vi "fake main magnet module.vi"(8 "Queue to UI":T10, 11 "Module queue":T10) -> ()   [LabVIEW 2022 SP3, in "Magnet module.lvlib"]
doc: "Magnet module controls: power supply unit (PSU/SMS) and temperature monitor (TM/LSC218).\nPSU controls mainly: switch heater and ramping of current which runs throught coil.\nTM controls temperature of switch, coil and cryostat.\nMessage for magnet is a cluster that contains: {(enum) Command , (variant) Data}\nFor simplifieing of documentation, the Command is noted as a name of instruction, and Data is represented by a requered datatype (mostly cluster) name.\nCommands:\nInitialize(Magnet Config Constants) - Sugesstion: Load configuration constants from configuration file.\nSet field (Set field{B, R, cr}) - B-field[T], R-ramp[A/s], cr - custom ramp[bool].\nSwitch mode(mode) - to persistant, or to ramping.\nBlackout() - undone functionality of emergency deenergizing.\nUpdate() - Important! This triggers update of data from instruments. Shoud occure in regular intervals as priority message.\nResponses:\nMagnet initialized ();\nTM revision(temperature monitor revision);\nMagnet init error(error);\nSetting field(Set Field{B, R, cr});\nWarning(string);\nSwitching to(mode);\nUpdate error(error);\nTM update(TM sensors);\nPSU update(PSU data);\nMagnet status();"
uses:
  Magnet module.lvlib
  Messenger service/Data types/Mailbox address.ctl
  <instrlib>/SMS 120/Public/PSU Status.ctl
  ctl/Cryostat temperature sensors.ctl
  ctl/Overall status.ctl
  ctl/SetField data.ctl
  ctl/Magnet mode public.ctl
  ctl/Actual magnet state.ctl
  ctl/Magnet mode.ctl
  ctl/RampingOutput.ctl
  ctl/Magnet config constants.ctl
  ctl/MagnetStates.ctl
  Messenger service/Data types/Module name.ctl
  ctl/TM Revision.ctl
  ctl/MSG to magnet.ctl
  ctl/Magnet Orders.ctl
  <instrlib>/SMS 120/Cryogenic Ltd SMSXXX.lvlib
  Messenger service/MessengerLib.lvlib
panel:
  in  "LSC218 sensors":T1={"First stage A [K]"=35.0, "Second stage A [K]"=4.0, "Firs stage B [K]"=33.0, "Second stage B [K]"=3.0, "Inner magnet [K]"=3.0, "Outer Magnet [K]"=3.5, "Switch [K]"=3.6, "Support plate [K]"=8.0, "Time stamp"=0.0} {"Time stamp" format="%<%H:%M:%S%2u\n%Y/%m/%d>T"}
  out "Magnet Constants":T2={"Switch resistant [K]"=5.0, "Switch superconducting [K]"=4.0, "First stage critical temperature [K]"=50.0, "Second stage critical temperature [K]"=5.0, "Inner magnet critical temperature [K]"=6.0, "Outer magnet critical temperature [K]"=5.0, "Field Constant [T/A]"=0.14911, "Maximum Current [A]"=107.3, "Maximum field [T]"=16.0, "Maximum source ramp [A/s]"=0.5, "Source precision [T]"=2e-05, "Ramp limits [A/s]"=[0.0506, 0.038, 0.0285, 0.0213, 0.0104], "Field limits [T]"=[3.0, 9.6, 13.3, 15.5, 16.0], "SMS"="", "LSC218"=""}
  out "Overall status":T3={"Desired"={"Field [T]"=0.0, "Ramp [T/s]"=0.0, "Custom Ramp?"=TRUE, "Mode"=enum."Persistant"}, "Actual"={"Mode"=enum."Persistant", "Ramping output"=enum."At Target", "Ready for change"=FALSE, "Switch heater"=FALSE, "Cooler Overheat"=FALSE, "Coil overheat"=FALSE, "Energized"=FALSE, "Output [T]"=0.0, "Field [T]"=0.0, "Ramp[T/s]"=0.0, "Switch\ntemperature [K]"=1.0, "Voltage [V]"=0.0, "Current direction"=FALSE}}
  out "Temperatures":T1[](array[typedef]) {"Time stamp" format="%<%H:%M:%S%2u\n%Y/%m/%d>T"}
  out "PSU Status Out":T9 {"Trip Current" format="%.3f"; "Trip Field" format="%.4f"; "Voltage" format="%.2f"; "Field Constant" format="%.6f"; "MID Setpoint (T)" format="%.4f"; "MID Setpoint (A)" format="%.3f"; "MAX Setpoint (T)" format="%.4f"; "MAX Setpoint (A)" format="%.3f"; "Heater Voltage" format="%.2f"; "V Limit (V)" format="%.2f"; "Ramp Rate (A/s)" format="%.3f"; "Output (A)" format="%.3f"; "Output (T)" format="%.4f"; "Persistent Current" format="%.3f"; "Persistent Field" format="%.4f"}
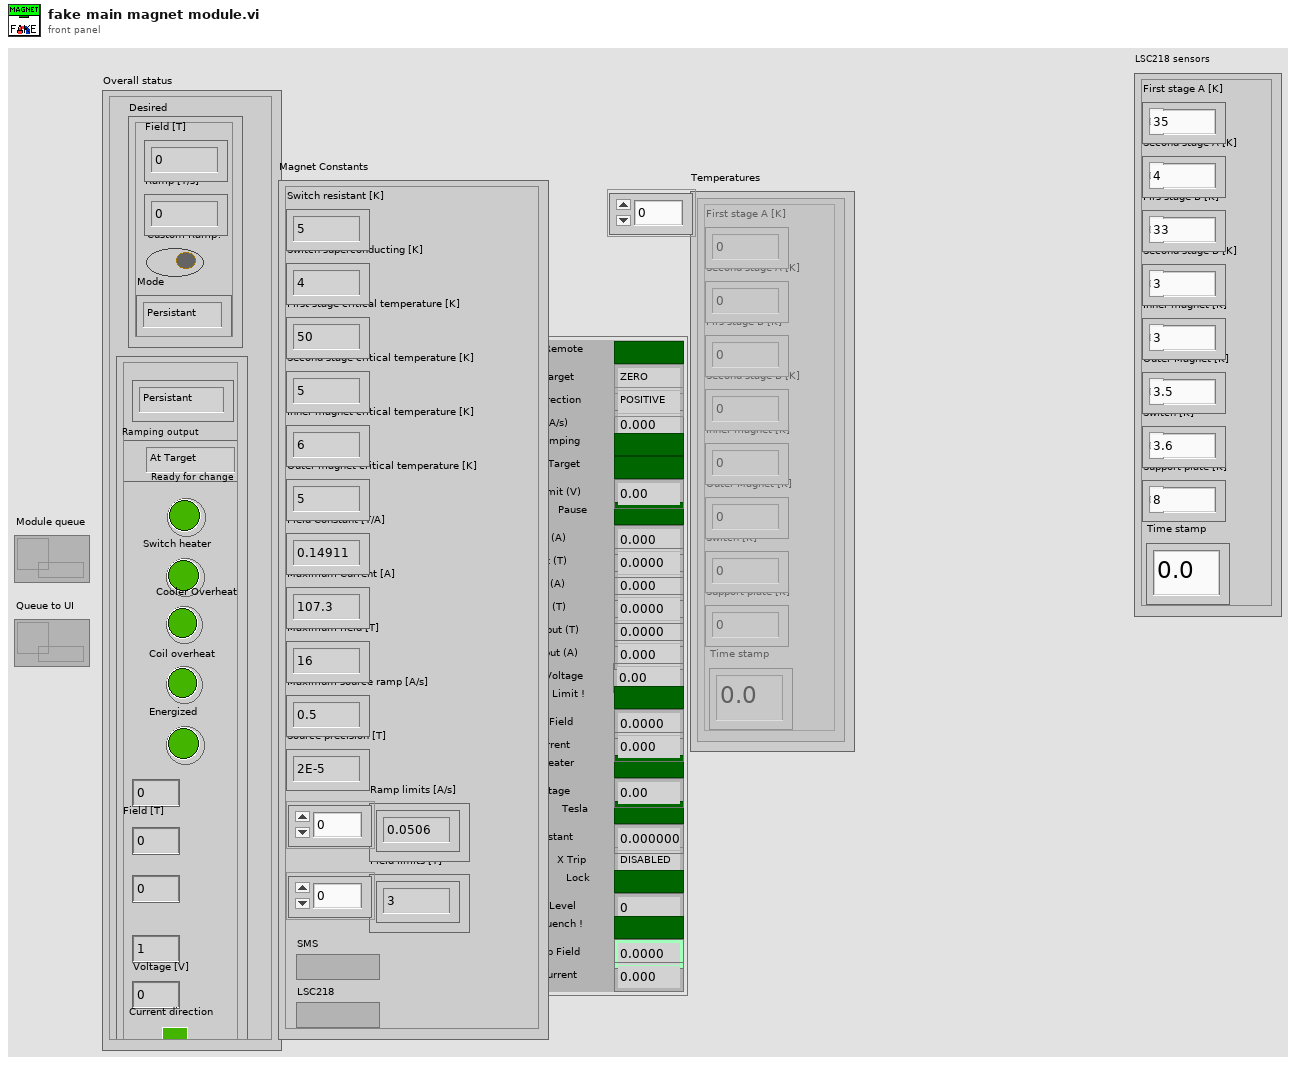
[diagram p1: front panel]
types:
  T1 = typedef "Magnet module.lvlib/Cryostat temperature sensors.ctl" = cluster{"First stage A [K]":dbl, "Second stage A [K]":dbl, "Firs stage B [K]":dbl, "Second stage B [K]":dbl, "Inner magnet [K]":dbl, "Outer Magnet [K]":dbl, "Switch [K]":dbl, "Support plate [K]":dbl, "Time stamp":dbl}
  T2 = typedef "Magnet module.lvlib/Magnet config constants.ctl" = cluster{"Switch resistant [K]":dbl, "Switch superconducting [K]":dbl, "First stage critical temperature [K]":dbl, "Second stage critical temperature [K]":dbl, "Inner magnet critical temperature [K]":dbl, "Outer magnet critical temperature [K]":dbl, "Field Constant [T/A]":dbl, "Maximum Current [A]":dbl, "Maximum field [T]":dbl, "Maximum source ramp [A/s]":dbl, "Source precision [T]":dbl, "Ramp limits [A/s]":dbl[], "Field limits [T]":dbl[], "SMS":refnum<visa-resource-name>, "LSC218":refnum<visa-resource-name>}
  T3 = typedef "Magnet module.lvlib/Overall status.ctl" = cluster{"Desired":T4, "Actual":T6}
  T4 = typedef "Magnet module.lvlib/SetField data.ctl" = cluster{"Field [T]":dbl, "Ramp [T/s]":dbl, "Custom Ramp?":bool, "Mode":T5}
  T5 = typedef "Magnet module.lvlib/Magnet mode public.ctl" = enum16{"Persistant", "Ramping"}
  T6 = typedef "Magnet module.lvlib/Actual magnet state.ctl" = cluster{"Mode":T7, "Ramping output":T8, "Ready for change":bool, "Switch heater":bool, "Cooler Overheat":bool, "Coil overheat":bool, "Energized":bool, "Output [T]":dbl, "Field [T]":dbl, "Ramp[T/s]":dbl, "Switch\ntemperature [K]":dbl, "Voltage [V]":dbl, "Current direction":bool}
  T7 = typedef "Magnet module.lvlib/Magnet mode.ctl" = enum16{"Persistant", "Switching", "Ramping", "Quenched"}
  T8 = typedef "Magnet module.lvlib/RampingOutput.ctl" = enum16{"At Target", "Go up", "Go down"}
  T9 = typedef "Cryogenic Ltd SMSXXX.lvlib/PSU Status.ctl" = cluster{"Ramp Target":enum16{"ZERO", "MID", "MAX"}, "Pause":bool, "Switch Heater":bool, "Persistent Field":dbl, "Persistent Current":dbl, "Tesla":bool, "Output (T)":dbl, "Output (A)":dbl, "X Trip":enum16{"DISABLED", "ENABLED", "ACTIVE"}, "Ramp Rate (A/s)":dbl, "V Limit (V)":dbl, "Heater Voltage":dbl, "MAX Setpoint (A)":dbl, "MAX Setpoint (T)":dbl, "MID Setpoint (A)":dbl, "MID Setpoint (T)":dbl, "Lock":bool, "Field Constant":dbl, "Remote":bool, "Direction":enum16{"POSITIVE", "NEGATIVE", "OPEN", "UNIPOLAR"}, "Helium Level":u16, "Quench !":bool, "Voltage":dbl, "V Limit !":bool, "Ramping":bool, "At Target":bool, "Trip Field":dbl, "Trip Current":dbl}
  T10 = typedef "MessengerLib.lvlib/Mailbox address.ctl" = refnum<queue>
  T11 = typedef "Magnet module.lvlib/MagnetStates.ctl" = enum16{"Initialize", "Regular check", "Check message", "Set Field", "Switch mode", "Restart", "Stop"}
  T12 = typedef "Magnet module.lvlib/MSG to magnet.ctl" = cluster{"Command":T13, "Data":variant}
  T13 = typedef "Magnet module.lvlib/Magnet Orders.ctl" = enum16{"Ignore", "Connect", "Update", "Switch mode", "Set field", "Stop ramping", "Equalize output", "Zero output", "Flip polarity", "Blackout", "Set timer", "Eval temperatures", "Disconnect"}
  T14 = typedef "Module name.ctl" = enum16{"Emty", "Magnet", "VTI", "Excitation", "Servo", "Acquisition", "Rotator", "Digitizer", "SMU2450", "Carousel", "Multimeter", "Tmp monitor", "Power monitor"}
  T15 = typedef "Magnet module.lvlib/TM Revision.ctl" = cluster{"Instr Serial Number":string, "Instr Driver Revision":string, "Instr Firmware Revision":string, "Instr Model Number":string}
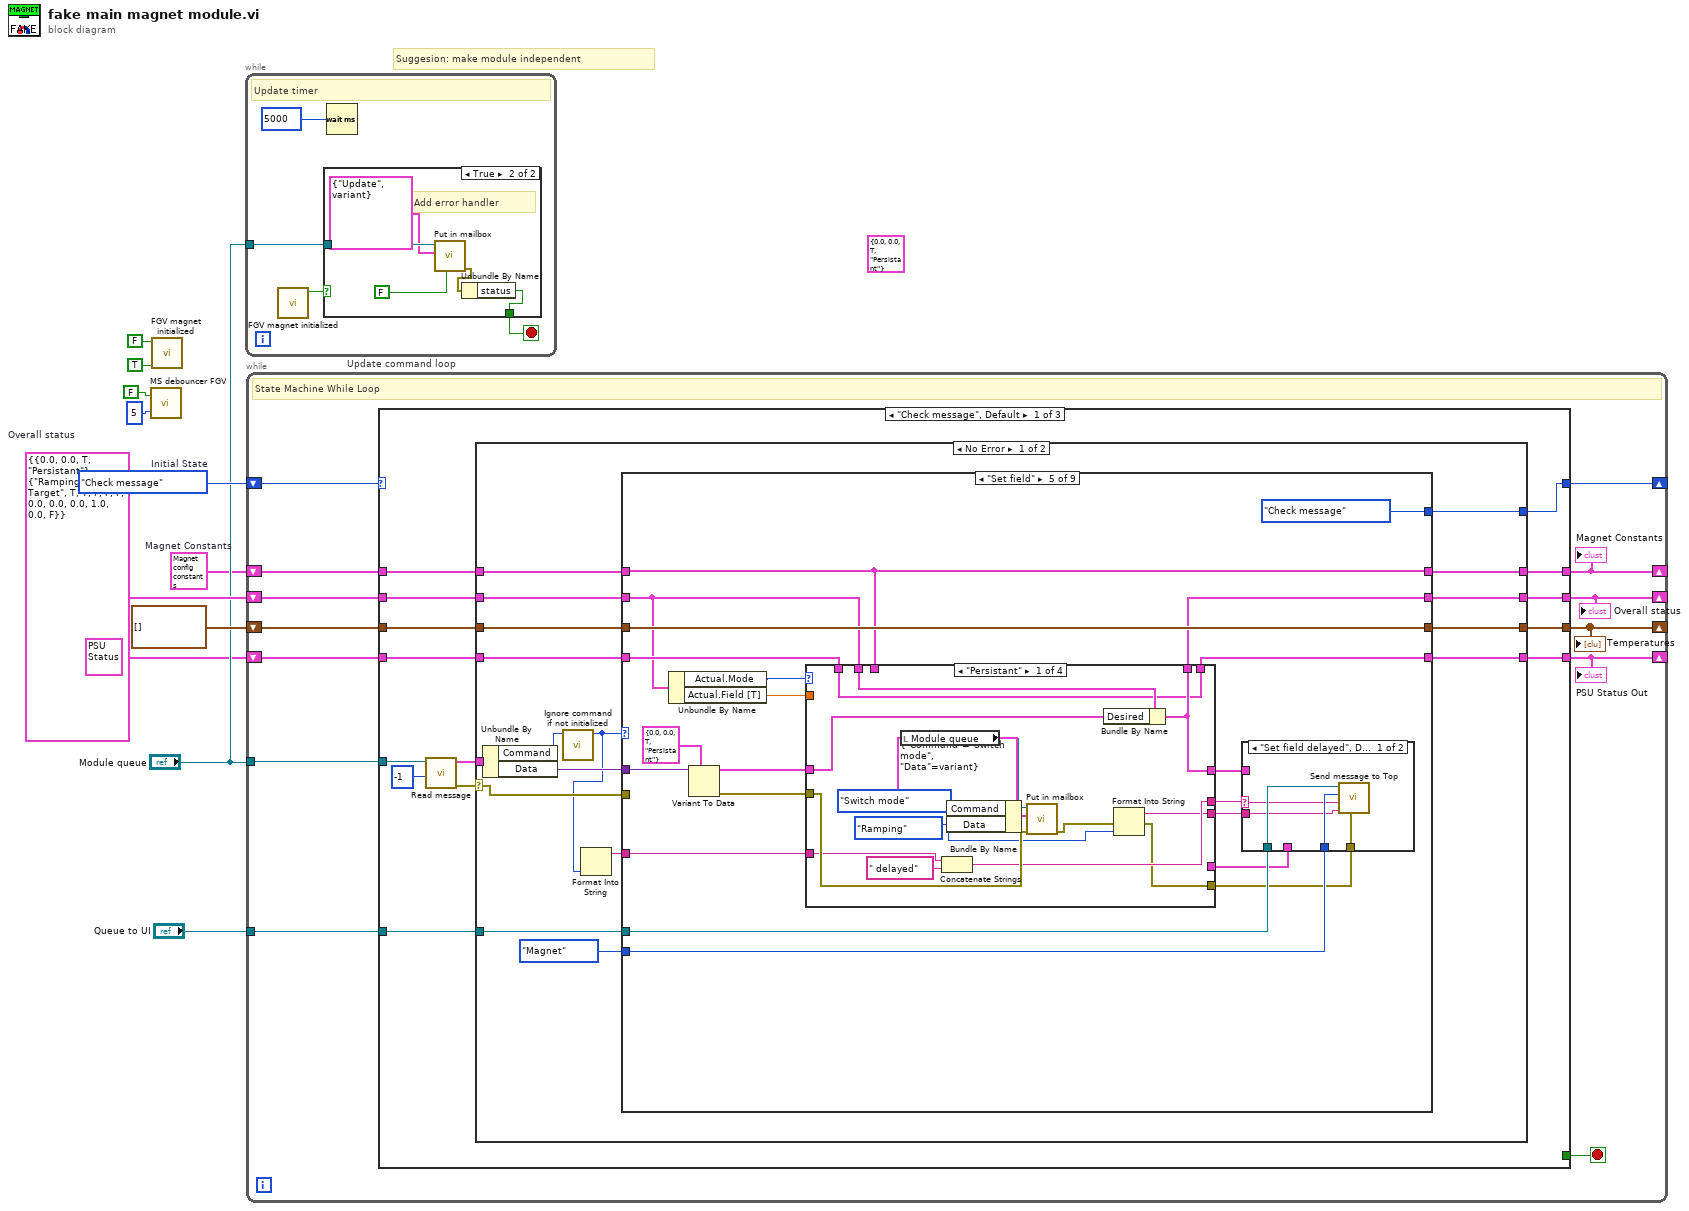
[diagram p0: block diagram]
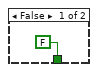
[diagram p2: hidden frame]
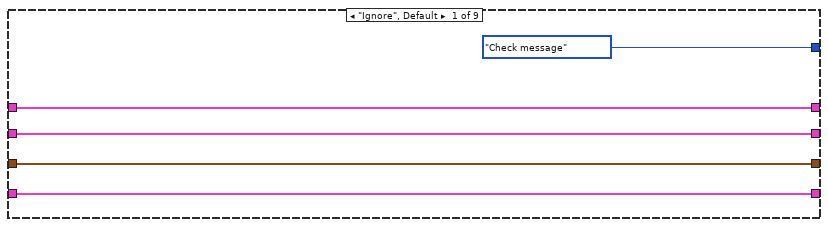
[diagram p3: hidden frame]
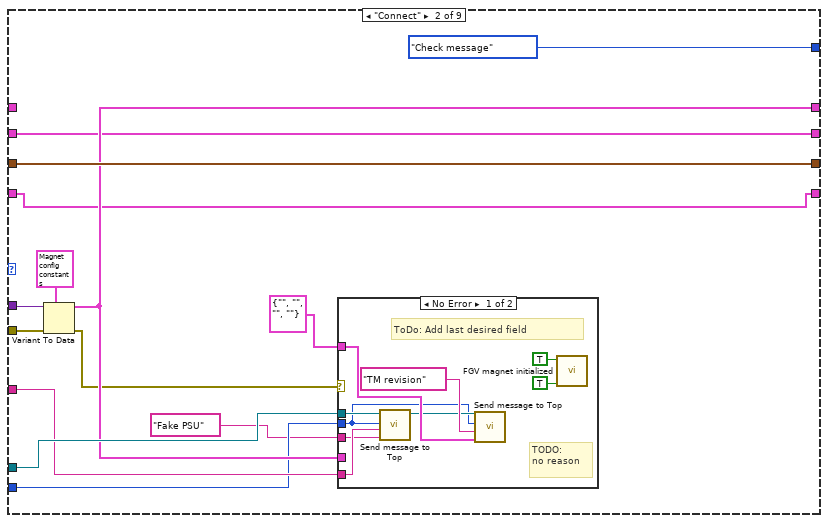
[diagram p4: hidden frame]
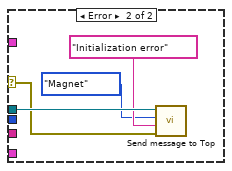
[diagram p5: hidden frame]
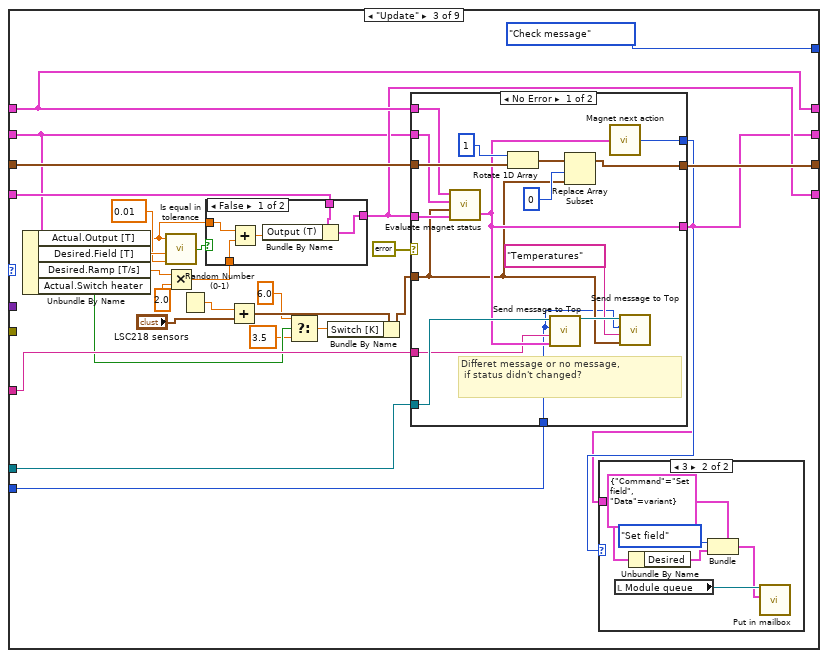
[diagram p6: hidden frame]
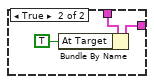
[diagram p8: hidden frame]
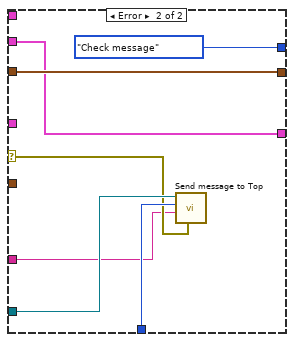
[diagram p9: hidden frame]
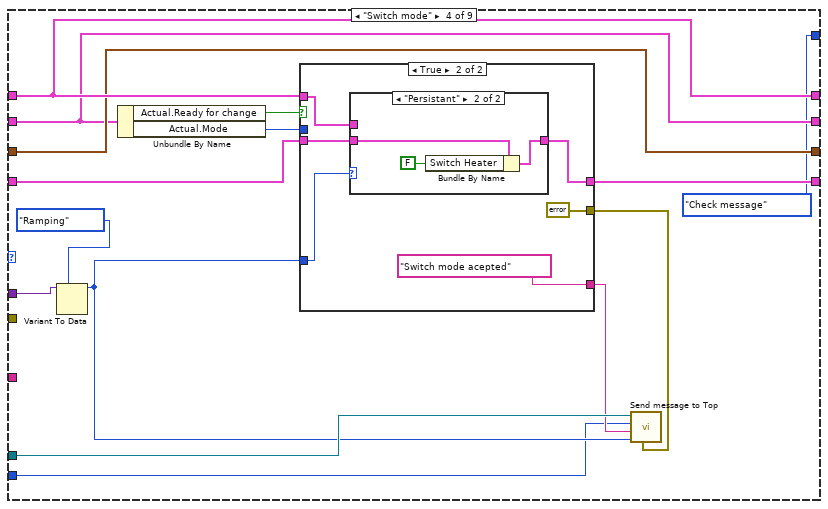
[diagram p10: hidden frame]
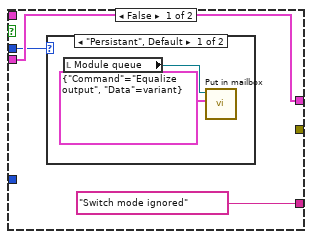
[diagram p11: hidden frame]
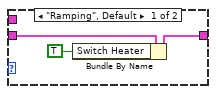
[diagram p13: hidden frame]
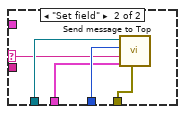
[diagram p14: hidden frame]
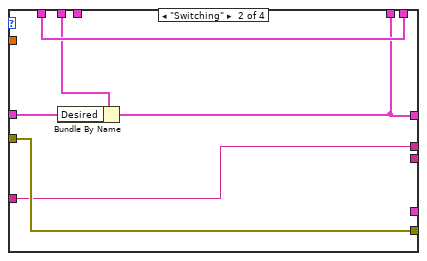
[diagram p15: hidden frame]
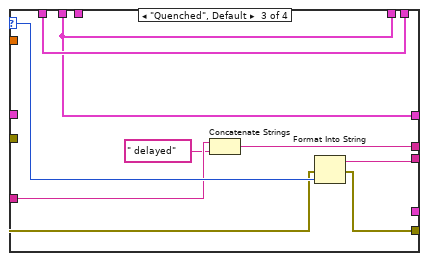
[diagram p16: hidden frame]
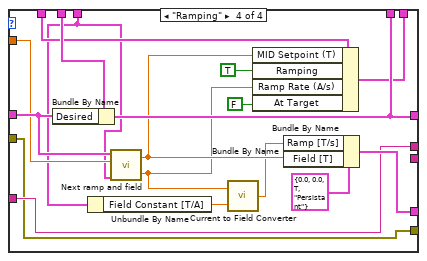
[diagram p17: hidden frame]
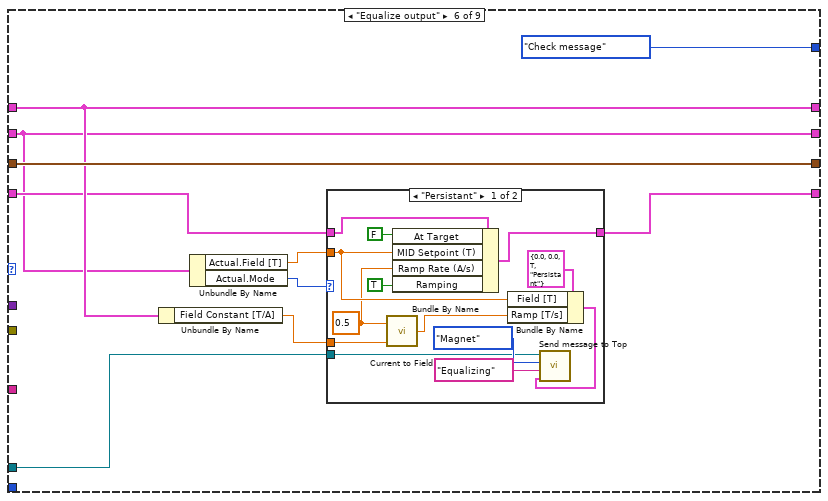
[diagram p18: hidden frame]
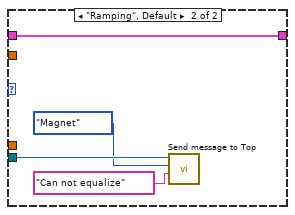
[diagram p19: hidden frame]
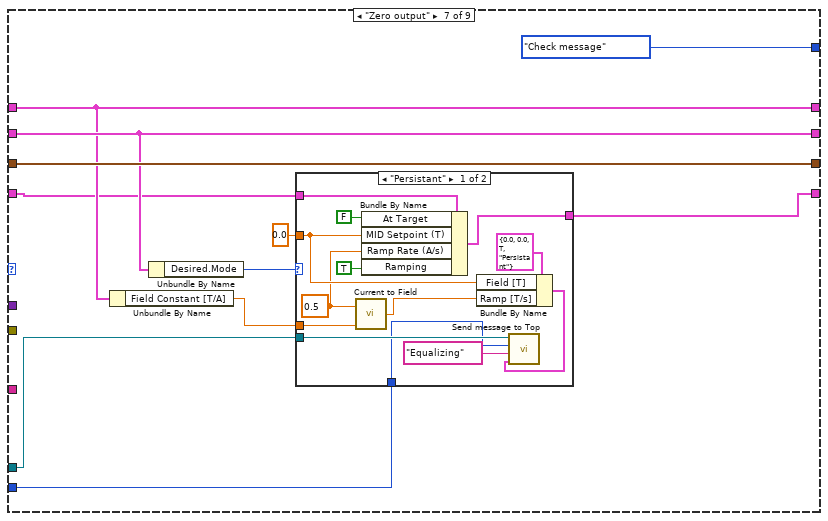
[diagram p20: hidden frame]
diagram:
  (unwired) T4 {"Field [T]"=0.0, "Ramp [T/s]"=0.0, "Custom Ramp?"=TRUE, "Mode"=enum."Persistant"} ("Set Field")
  w1 = T2 {"Switch resistant [K]"=5.0, "Switch superconducting [K]"=4.0, "First stage critical temperature [K]"=50.0, "Second stage critical temperature [K]"=5.0, "Inner magnet critical temperature [K]"=6.0, "Outer magnet critical temperature [K]"=5.0, "Field Constant [T/A]"=0.14911, "Maximum Current [A]"=107.3, "Maximum field [T]"=16.0, "Maximum source ramp [A/s]"=0.5, "Source precision [T]"=2e-05, "Ramp limits [A/s]"=[0.0506, 0.038, 0.0285, 0.0213, 0.0104], "Field limits [T]"=[3.0, 9.6, 13.3, 15.5, 16.0], "SMS"="COM3", "LSC218"="COM1"}  # Magnet Constants
  w10 = T3 {"Desired"={"Field [T]"=0.0, "Ramp [T/s]"=0.0, "Custom Ramp?"=TRUE, "Mode"=enum."Persistant"}, "Actual"={"Mode"=enum."Ramping", "Ramping output"=enum."At Target", "Ready for change"=TRUE, "Switch heater"=TRUE, "Cooler Overheat"=FALSE, "Coil overheat"=FALSE, "Energized"=FALSE, "Output [T]"=0.0, "Field [T]"=0.0, "Ramp[T/s]"=0.0, "Switch\ntemperature [K]"=1.0, "Voltage [V]"=0.0, "Current direction"=FALSE}}  # Overall status
  w11 = MagnetStates."Check message"  # Initial State
  # "Suggesion: make module independent"
  n1 = call "MS debouncer FGV.vi"("Iterations"=5, "At target?"=FALSE ("On target?")) -> ()  [unwired: 1 out]
  n2 = call "FGV magnet initialized.vi"("Write?(F)"=TRUE, "Initialized in"=FALSE) -> ()  [unwired: 9 in, 1 out]
  n3 = while "Update command loop" {
    tunnel: "Module queue" -> [w14]
    stop <- w12 stop-if-true
    # "Update timer"
    n4 = call "FGV magnet initialized.vi"() -> ("Initialized out"=w13:bool)  [unwired: 11 in]
    n5 = case shown="True" w13 {
      tunnel: w14 -> [_ w21]
      tunnel: [FALSE w18] -> w12
      frame False {
      }
      frame True {
        # "Add error handler"
        n6 = call "Put in mailbox.vi"("Priority? (F)"=FALSE ("Priority?"), "Message"=T12 {"Command"=enum."Update", "Data"=variant(enum16{"Ramping", "Perzistant"} enum."Ramping")} ("MSG to magnet"), "Queue in"=w21) -> ("error out"=w19:errorcluster)  [unwired: 6 in, 2 out]
        n7 = Unbundle By Name(w19) -> ("status"=w18:bool)
      }
    }
    n8 = Wait (ms)(milliseconds to wait=u32 5000) -> ()  [unwired: 1 out]
  }
  n9 = while {
    shift-right: [w23] -> _
    shift-left: w11 -> [w34]
    tunnel: "Module queue" -> [w32]
    tunnel: "Queue to UI" -> [w31]
    shift-right: [w26] -> _
    shift-left: w10 -> [w27]
    shift-right: [w28] -> _
    shift-left: T1[] [] ("Temperatures") -> [w29]
    shift-right: [w25] -> _
    shift-left: T9 {"Ramp Target"=enum."ZERO", "Pause"=FALSE, "Switch Heater"=FALSE, "Persistent Field"=0.0, "Persistent Current"=0.0, "Tesla"=FALSE, "Output (T)"=0.0, "Output (A)"=0.0, "X Trip"=enum."DISABLED", "Ramp Rate (A/s)"=0.0, "V Limit (V)"=0.0, "Heater Voltage"=0.0, "MAX Setpoint (A)"=0.0, "MAX Setpoint (T)"=0.0, "MID Setpoint (A)"=0.0, "MID Setpoint (T)"=0.0, "Lock"=FALSE, "Field Constant"=0.0, "Remote"=FALSE, "Direction"=enum."POSITIVE", "Helium Level"=0, "Quench !"=FALSE, "Voltage"=0.0, "V Limit !"=FALSE, "Ramping"=FALSE, "At Target"=FALSE, "Trip Field"=0.0, "Trip Current"=0.0} ("PSU Status Out") -> [w24]
    shift-right: [w30] -> _
    shift-left: w1 -> [w22]
    stop <- w33 stop-if-true
    # "State Machine While Loop"
    n10 = case "State Machine Case Structure" shown="\"Check message\", Default" w34 {
      tunnel: [_ w374 _] -> w33
      tunnel: w32 -> [w35 _ _]
      tunnel: [w45 MagnetStates."Stop" ("Initial State") MagnetStates."Initialize" ("Initial State")] -> w23
      tunnel: w31 -> [w47 w371 _]
      tunnel: w27 -> [w44 w363 w376]
      tunnel: w22 -> [w43 w361 w377]
      tunnel: [w42 w361 w377] -> w30
      tunnel: w29 -> [w41 w372 w378]
      tunnel: [w40 w372 w378] -> w28
      tunnel: [w38 w363 w376] -> w26
      tunnel: [w37 w362 w375] -> w25
      tunnel: w24 -> [w36 w362 w375]
      frame "Check message", Default {
        # "Wait for Event - An Event Structure is used to monitor the user interface for events. In each frame of the Event Structure, the next state of the state machine is specified based on which button was pressed."
        n11 = call "Read message.vi"("timeout in ms (10)"=-1 ("timeout in ms (-1)"), "Module queue ref"=w35) -> ("error out"=w39:errorcluster, "MSG to magnet"=w46:T12)  [unwired: 8 in]
        n12 = case shown="No Error" w39 {
          selector: w39 -> [w52 _]
          tunnel: w47 -> [w65 _]
          tunnel: w46 -> [w57 _]
          tunnel: [w64 w359] -> w38
          tunnel: [w63 MagnetStates."Check message" ("Initial State")] -> w45
          tunnel: w44 -> [w62 w359]
          tunnel: w43 -> [w61 w360]
          tunnel: [w60 w360] -> w42
          tunnel: w41 -> [w59 w358]
          tunnel: [w58 w358] -> w40
          tunnel: [w55 w356] -> w37
          tunnel: w36 -> [w54 w356]
          frame No Error {
            n13 = Unbundle By Name(w57) -> ("Command"=w56:T13, "Data"=w53:variant)
            n14 = call "Ignore command if not initialized.vi"("Command in"=w56) -> ("Command out"=w50:T13)  [unwired: 10 in]
            n15 = Format Into String(w50) -> (resulting string=w49:string)  [unwired: 3 in, 1 out]
            n16 = case shown="\"Set field\"" w50 {
              tunnel: w65 -> [_ w83 w124 w177 w211 w277 w306 _ w346]
              tunnel: [w70 w73 w106 w173 w207 w276 w309 w333 w347] -> w64
              tunnel: [MagnetStates."Check message" ("Initial State") MagnetStates."Check message" ("Initial State") MagnetStates."Check message" ("Next state") MagnetStates."Check message" ("t") MagnetStates."Check message" ("t") MagnetStates."Check message" ("Initial State") MagnetStates."Check message" ("Initial State") MagnetStates."Check message" ("Initial State") MagnetStates."Stop" ("Initial State")] -> w63
              tunnel: w62 -> [w70 w73 w115 w173 w206 w276 w309 w333 w347]
              tunnel: w61 -> [w69 _ w125 w175 w197 w281 w308 w336 w345]
              tunnel: [w69 w78 w125 w175 w197 w281 w308 w336 w345] -> w60
              tunnel: w59 -> [w68 w82 w123 w174 w214 w282 w310 w335 w354]
              tunnel: [w68 w82 w122 w174 w214 w282 w310 w335 w354] -> w58
              tunnel: [w66 w72 w116 w171 w209 w278 w302 w334 w353] -> w55
              tunnel: w54 -> [w66 w72 w117 w172 w210 w279 w303 w334 w353]
              tunnel: w53 -> [_ w81 _ w169 w212 _ _ w331 _]
              tunnel: w52 -> [_ w79 _ _ _ _ _ _ _]
              tunnel: Module_name."Magnet" ("Module") -> [_ w76 w121 w166 w205 _ w305 _ w343]
              tunnel: w49 -> [_ w77 w119 _ w198 _ _ _ w344]
              frame "Ignore", Default {
              }
              frame "Connect" {
                n17 = Variant To Data(error in=w79, type=T2 {"Switch resistant [K]"=5.0, "Switch superconducting [K]"=4.0, "First stage critical temperature [K]"=50.0, "Second stage critical temperature [K]"=5.0, "Inner magnet critical temperature [K]"=6.0, "Outer magnet critical temperature [K]"=5.0, "Field Constant [T/A]"=0.14911, "Maximum Current [A]"=107.3, "Maximum field [T]"=16.0, "Maximum source ramp [A/s]"=0.5, "Source precision [T]"=2e-05, "Ramp limits [A/s]"=[0.0506, 0.038, 0.0285, 0.0213, 0.0104], "Field limits [T]"=[3.0, 9.6, 13.3, 15.5, 16.0], "SMS"="", "LSC218"=""} ("Magnet Config Constants"), Variant=w81) -> (data=w78:T2, error out=w71:errorcluster)
                n18 = case shown="No Error" w71 {
                  selector: w71 -> [_ w96]
                  tunnel: w83 -> [w89 w97]
                  tunnel: T15 {"Instr Serial Number"="", "Instr Driver Revision"="", "Instr Firmware Revision"="", "Instr Model Number"=""} ("TM Revision") -> [w90 _]
                  tunnel: "Fake PSU" ("Initial message") -> [w85 _]
                  tunnel: w78 -> [_ _]
                  tunnel: w77 -> [w87 _]
                  tunnel: w76 -> [w86 _]
                  frame No Error {
                    # "TODO:\nno reason"
                    # "ToDo: Add last desired field"
                    n19 = call "Send message to Top.vi"("Data"=w85, "Response"=w87, "Module"=w86, "Mailbox address in"=w89) -> ("Mailbox address out"=w88:T10)  [unwired: 6 in, 1 out]
                    n20 = call "Send message to Top.vi"("Data"=w90, "Response"="TM revision" ("Name"), "Module"=w86, "Mailbox address in"=w88) -> ()  [unwired: 6 in, 2 out]
                    n21 = call "FGV magnet initialized.vi"("Write?(F)"=TRUE, "Initialized in"=TRUE) -> ()  [unwired: 9 in, 1 out]
                  }
                  frame Error {
                    n22 = call "Send message to Top.vi"("Data"=w96, "Response"="Initialization error" ("Command"), "Module"=Module_name."Magnet", "Mailbox address in"=w97) -> ()  [unwired: 6 in, 2 out]
                  }
                }
              }
              frame "Update" {
                n23 = Unbundle By Name(w115) -> ("Actual.Output [T]"=w110:dbl, "Desired.Field [T]"=w114:dbl, "Desired.Ramp [T/s]"=w112:dbl, "Actual.Switch heater"=w100:bool)
                n24 = call "Is equal in tolerance.vi"("Absolut tolerance"=0.01, "Reference value"=w114, "Input value"=w110) -> ("Is in range"=w108:bool)  [unwired: 1 in]
                n25 = Multiply(x=w112, y=2.0) -> (x*y=w109:dbl)
                n26 = Random Number (0-1)() -> (number: 0 to 1=w103:dbl)
                n27 = case shown="False" w108 {
                  tunnel: w117 -> [w136 w139]
                  tunnel: [w135 w138] -> w116
                  tunnel: w110 -> [w134 _]
                  tunnel: w109 -> [w133 _]
                  frame False {
                    n28 = Add(x=w134, y=w133) -> (x+y=w132:dbl)
                    n29 = Bundle By Name(cluster=w136, "Output (T)"=w132) -> (w135:T9)
                  }
                  frame True {
                    n30 = Bundle By Name(cluster=w139, "At Target"=TRUE) -> (w138:T9)
                  }
                }
                n31 = Add(x=w103, y="LSC218 sensors") -> (x+y=w104:T1)
                n32 = Select(t=6.0, s=w100, f=3.5) -> (s? t:f=w101:dbl)
                n33 = Bundle By Name(cluster=w104, "Switch [K]"=w101) -> (w102:T1)
                n34 = case shown="No Error" errorcluster {"status"=FALSE, "code"=0, "source"=""} ("error IO") {
                  selector: errorcluster {"status"=FALSE, "code"=0, "source"=""} ("error IO") -> [_ w157]
                  tunnel: w124 -> [w150 w161]
                  tunnel: w102 -> [w142 _]
                  tunnel: w116 -> [w149 _]
                  tunnel: [w146 w159] -> w106
                  tunnel: w123 -> [w153 w162]
                  tunnel: [w151 w162] -> w122
                  tunnel: w125 -> [w148 _]
                  tunnel: [w147 MagnetStates."Check message" ("Next state")] -> w107
                  tunnel: w115 -> [w145 w159]
                  tunnel: w121 -> [w140 w158]
                  tunnel: w119 -> [w144 w156]
                  frame No Error {
                    # "Differet message or no message,\n if status didn't changed?"
                    n35 = call "Evaluate magnet status.vi"("PSU Status in"=w149, "LSC218 sensors"=w142, "Overall status in"=w145, "Magnet Constants"=w148) -> ("Overall status out"=w146:T3)  [unwired: 1 in]
                    n36 = Rotate 1D Array(1:w153, 2:1 ("n")) -> (0:w154:T1[])
                    n37 = call "Send message to Top.vi"("Data"=w146, "Response"=w144, "Module"=w140, "Mailbox address in"=w150) -> ("Mailbox address out"=w143:T10)  [unwired: 6 in, 1 out]
                    n38 = Replace Array Subset(array=w154, new element=w142, index=0) -> (w151:T1[])
                    n39 = call "Magnet next action.vi"("Overall status in"=w146) -> ("Command out"=w147:T13)  [unwired: 3 in, 1 out]
                    n40 = call "Send message to Top.vi"("Data"=w142, "Response"="Temperatures", "Module"=w140, "Mailbox address in"=w143) -> ()  [unwired: 6 in, 2 out]
                  }
                  frame Error {
                    n41 = call "Send message to Top.vi"("Error in (no error)"=w157, "Response"=w156, "Module"=w158, "Mailbox address in"=w161) -> ()  [unwired: 6 in, 2 out]
                  }
                }
                n42 = case shown="3" w107 {
                  tunnel: w106 -> [_ w127]
                  frame 2, Default {
                  }
                  frame 3 {
                    n43 = local read "Module queue"() -> (w131:T10)
                    n44 = Unbundle By Name(w127) -> ("Desired"=w128:T4)
                    n45 = Bundle(cluster=T12 {"Command"=enum."Set field", "Data"=variant} ("MSG to magnet"), "Command"=Magnet_Orders."Set field" ("Order"), "Data"=w128) -> (w126:T12)
                    n46 = call "Put in mailbox.vi"("Message"=w126, "Queue in"=w131) -> ()  [unwired: 7 in, 3 out]
                  }
                }
              }
              frame "Switch mode" {
                n47 = Variant To Data(type=Magnet_mode_public."Ramping" ("Operation mode"), Variant=w169) -> (data=w168:T5)  [unwired: 1 in, 1 out]
                n48 = Unbundle By Name(w173) -> ("Actual.Ready for change"=w176:bool, "Actual.Mode"=w164:T7)
                n49 = case shown="True" w176 {
                  tunnel: w168 -> [_ w187]
                  tunnel: w175 -> [_ w188]
                  tunnel: w172 -> [w180 w186]
                  tunnel: [w180 w185] -> w171
                  tunnel: ["Switch mode ignored" ("Name") "Switch mode acepted" ("Name")] -> w170
                  tunnel: w164 -> [w178 _]
                  tunnel: [_ errorcluster {"status"=FALSE, "code"=0, "source"=""} ("Error out")] -> w163
                  frame False {
                    n50 = case shown="\"Persistant\", Default" w178 {
                      frame "Persistant", Default {
                        n51 = local read "Module queue"() -> (w181:T10)
                        n52 = call "Put in mailbox.vi"("Message"=T12 {"Command"=enum."Equalize output", "Data"=variant(enum16{"Ramping", "Perzistant"} enum."Ramping")} ("MSG to magnet"), "Queue in"=w181) -> ()  [unwired: 7 in, 3 out]
                      }
                      frame "Ramping" {
                      }
                    }
                  }
                  frame True {
                    n53 = case shown="\"Persistant\"" w187 {
                      tunnel: w188 -> [_ _]
                      tunnel: w186 -> [w191 w193]
                      tunnel: [w190 w194] -> w185
                      frame "Ramping", Default {
                        n54 = Bundle By Name(cluster=w191, "Switch Heater"=TRUE) -> (w190:T9)
                      }
                      frame "Persistant" {
                        n55 = Bundle By Name(cluster=w193, "Switch Heater"=FALSE) -> (w194:T9)
                      }
                    }
                  }
                }
                n56 = call "Send message to Top.vi"("Error in (no error)"=w163, "Data"=w168, "Response"=w170, "Module"=w166, "Mailbox address in"=w177) -> ()  [unwired: 5 in, 2 out]
              }
              frame "Set field" {
                n57 = Unbundle By Name(w206) -> ("Actual.Mode"=w215:T7, "Actual.Field [T]"=w196:dbl)
                n58 = Variant To Data(type=T4 {"Field [T]"=0.0, "Ramp [T/s]"=0.0, "Custom Ramp?"=TRUE, "Mode"=enum."Persistant"} ("Set Field"), Variant=w212) -> (data=w208:T4, error out=w204:errorcluster)  [unwired: 1 in]
                n59 = case shown="\"Persistant\"" w215 {
                  selector: w215 -> [_ _ w252 _]
                  tunnel: w206 -> [w241 w245 w255 w271]
                  tunnel: w197 -> [_ _ _ w259]
                  tunnel: w210 -> [w238 w247 w256 w266]
                  tunnel: [w238 w247 w256 w265] -> w209
                  tunnel: w208 -> [w239 w244 _ w273]
                  tunnel: [w240 w243 w255 w270] -> w207
                  tunnel: w204 -> [w234 w246 w251 w258]
                  tunnel: [w240 w243 w255 w270] -> w203
                  tunnel: [w230 w242 w254 w268] -> w202
                  tunnel: [w226 w246 w250 w258] -> w201
                  tunnel: [_ _ _ w269] -> w200
                  tunnel: w198 -> [w232 w242 w249 w268]
                  tunnel: w196 -> [_ _ _ w267]
                  tunnel: [w229 _ w253 _] -> w195
                  frame "Persistant" {
                    w231 = Magnet_Orders."Switch mode" ("Order")
                    n60 = local read "Module queue"() -> (w235:T10)
                    n61 = Concatenate Strings(w232, " delayed" ("string")) -> (w230:string)
                    n62 = Bundle By Name(cluster=T12 {"Command"=enum."Switch mode", "Data"=variant(enum16{"Ramping", "Perzistant"} enum."Ramping")} ("MSG to magnet"), "Command"=w231, "Data"=Magnet_mode_public."Ramping" ("Operation mode")) -> (w237:T12)
                    n63 = call "Put in mailbox.vi"("error in (no error)"=w234, "Message"=w237, "Queue in"=w235) -> ("error out"=w227:errorcluster)  [unwired: 6 in, 2 out]
                    n64 = Bundle By Name(cluster=w241, "Desired"=w239) -> (w240:T3)
                    n65 = Format Into String(error in=w227, w231) -> (resulting string=w229:string, error out=w226:errorcluster)  [unwired: 2 in]
                  }
                  frame "Switching" {
                    n66 = Bundle By Name(cluster=w245, "Desired"=w244) -> (w243:T3)
                  }
                  frame "Quenched", Default {
                    n67 = Concatenate Strings(w249, " delayed" ("string")) -> (w254:string)
                    n68 = Format Into String(error in=w251, w252) -> (resulting string=w253:string, error out=w250:errorcluster)  [unwired: 2 in]
                  }
                  frame "Ramping" {
                    n69 = Bundle By Name(cluster=w271, "Desired"=w273) -> (w270:T3)
                    n70 = Unbundle By Name(w259) -> ("Field Constant [T/A]"=w262:dbl)
                    n71 = call "Next ramp and field.vi"("Magnet Constants in"=w259, "Actual field [T]"=w267, "Desired"=w273) -> ("Ramp to set [A/s]"=w261:dbl, "Field to set [T]"=w263:dbl)  [unwired: 1 in]
                    n72 = call "Current to Field Converter.vi"("Field constant [T/A]"=w262, "Current in [A]"=w261) -> ("Field out [T]"=w260:dbl)
                    n73 = Bundle By Name(cluster=w266, "MID Setpoint (T)"=w263, "Ramping"=TRUE, "Ramp Rate (A/s)"=w261, "At Target"=FALSE) -> (w265:T9)
                    n74 = Bundle By Name(cluster=T4 {"Field [T]"=0.0, "Ramp [T/s]"=0.0, "Custom Ramp?"=TRUE, "Mode"=enum."Persistant"} ("Desired"), "Ramp [T/s]"=w260, "Field [T]"=w263) -> (w269:T4)
                  }
                }
                n75 = case shown="\"Set field delayed\", Default" w202 {
                  selector: w202 -> [w218 w222]
                  tunnel: w211 -> [w220 w225]
                  tunnel: w205 -> [w219 w224]
                  tunnel: w201 -> [w217 w223]
                  tunnel: w203 -> [_ _]
                  tunnel: w200 -> [_ w221]
                  tunnel: w195 -> [w216 _]
                  frame "Set field delayed", Default {
                    n76 = call "Send message to Top.vi"("Error in (no error)"=w217, "Data"=w216, "Response"=w218, "Module"=w219, "Mailbox address in"=w220) -> ()  [unwired: 5 in, 2 out]
                  }
                  frame "Set field" {
                    n77 = call "Send message to Top.vi"("Error in (no error)"=w223, "Data"=w221, "Response"=w222, "Module"=w224, "Mailbox address in"=w225) -> ()  [unwired: 5 in, 2 out]
                  }
                }
              }
              frame "Equalize output" {
                n78 = Unbundle By Name(w281) -> ("Field Constant [T/A]"=w280:dbl)
                n79 = Unbundle By Name(w276) -> ("Actual.Field [T]"=w274:dbl, "Actual.Mode"=w275:T7)
                n80 = case shown="\"Persistant\"" w275 {
                  tunnel: w280 -> [w286 _]
                  tunnel: w274 -> [w287 _]
                  tunnel: w279 -> [w291 w300]
                  tunnel: [w290 w300] -> w278
                  tunnel: w277 -> [w294 w299]
                  frame "Persistant" {
                    w284 = 0.5 ("Ramp to set [A/s]")
                    n81 = call "Current to Field.vi"("Field constant [T/A]"=w286, "Current in [A]"=w284) -> ("Field out [T]"=w285:dbl)
                    n82 = Bundle By Name(cluster=w291, "At Target"=FALSE, "MID Setpoint (T)"=w287, "Ramp Rate (A/s)"=w284, "Ramping"=TRUE) -> (w290:T9)
                    n83 = Bundle By Name(cluster=T4 {"Field [T]"=0.0, "Ramp [T/s]"=0.0, "Custom Ramp?"=TRUE, "Mode"=enum."Persistant"} ("Desired"), "Field [T]"=w287, "Ramp [T/s]"=w285) -> (w292:T4)
                    n84 = call "Send message to Top.vi"("Data"=w292, "Response"="Equalizing", "Module"=Module_name."Magnet", "Mailbox address in"=w294) -> ()  [unwired: 6 in, 2 out]
                  }
                  frame "Ramping", Default {
                    n85 = call "Send message to Top.vi"("Response"="Can not equalize", "Module"=Module_name."Magnet", "Mailbox address in"=w299) -> ()  [unwired: 7 in, 2 out]
                  }
                }
              }
              frame "Zero output" {
                n86 = Unbundle By Name(w308) -> ("Field Constant [T/A]"=w307:dbl)
                n87 = Unbundle By Name(w309) -> ("Desired.Mode"=w304:T5)
                n88 = case shown="\"Persistant\"" w304 {
                  tunnel: w307 -> [w315 _]
                  tunnel: 0.0 ("Field [T]") -> [w316 _]
                  tunnel: w303 -> [w320 w328]
                  tunnel: [w319 w328] -> w302
                  tunnel: w306 -> [w323 w327]
                  tunnel: w305 -> [w312 _]
                  frame "Persistant" {
                    w313 = 0.5 ("Ramp to set [A/s]")
                    n89 = call "Current to Field.vi"("Field constant [T/A]"=w315, "Current in [A]"=w313) -> ("Field out [T]"=w314:dbl)
                    n90 = Bundle By Name(cluster=w320, "At Target"=FALSE, "MID Setpoint (T)"=w316, "Ramp Rate (A/s)"=w313, "Ramping"=TRUE) -> (w319:T9)
                    n91 = Bundle By Name(cluster=T4 {"Field [T]"=0.0, "Ramp [T/s]"=0.0, "Custom Ramp?"=TRUE, "Mode"=enum."Persistant"} ("Desired"), "Field [T]"=w316, "Ramp [T/s]"=w314) -> (w321:T4)
                    n92 = call "Send message to Top.vi"("Data"=w321, "Response"="Equalizing", "Module"=w312, "Mailbox address in"=w323) -> ()  [unwired: 6 in, 2 out]
                  }
                  frame "Ramping", Default {
                    n93 = call "Send message to Top.vi"("Response"="Can not equalize", "Module"=Module_name."Magnet", "Mailbox address in"=w327) -> ()  [unwired: 7 in, 2 out]
                  }
                }
              }
              frame "Blackout" {
                n94 = Variant To Data(type=TRUE ("Actual.Energized"), Variant=w331) -> (data=w329:bool)  [unwired: 1 in, 1 out]
                n95 = Unbundle By Name(w333) -> ("Actual.Energized"=w337:bool)
                n96 = And(x=w337, y=w329) -> (x .and. y?=w338:bool)
                n97 = case shown="True" w338 {
                  frame True {
                    n98 = local read "Module queue"() -> (w342:T10)
                    n99 = Bundle By Name(cluster=T12 {"Command"=enum."Set field", "Data"=variant} ("MSG to magnet"), "Data"=T4 {"Field [T]"=0.0, "Ramp [T/s]"=0.0, "Custom Ramp?"=FALSE, "Mode"=enum."Persistant"} ("Set Field")) -> (w341:T12)
                    n100 = call "Put in mailbox.vi"("Message"=w341, "Queue in"=w342) -> ()  [unwired: 7 in, 3 out]
                  }
                  frame False {
                  }
                }
              }
              frame "Set timer" {
                n101 = call "Send message to Top.vi"("Data"=w345, "Response"="TM closed", "Module"=Module_name."Magnet", "Mailbox address in"=w346) -> ("Mailbox address out"=w348:T10)  [unwired: 6 in, 1 out]
                n102 = call "FGV magnet initialized.vi"("Write?(F)"=TRUE, "Initialized in"=FALSE) -> ()  [unwired: 9 in, 1 out]
                n103 = call "Send message to Top.vi"("Data"=w347, "Response"=w344, "Module"=w343, "Mailbox address in"=w348) -> ()  [unwired: 6 in, 2 out]
              }
            }
          }
          frame Error {
            # "add error handler?"
          }
        }
      }
      frame "Stop" {
        w374 = TRUE  # Stop the Loop
        # "Stop - Stop the VI. This is the only state that specifies a TRUE value for the loop conditional terminal."
        n104 = call "Send message to Top.vi"("Data"=w361, "Response"="TM closed", "Module"=Module_name."Magnet", "Mailbox address in"=w371) -> ("Mailbox address out"=w366:T10)  [unwired: 6 in, 1 out]
        n105 = call "FGV magnet initialized.vi"("Write?(F)"=TRUE, "Initialized in"=FALSE) -> ()  [unwired: 9 in, 1 out]
        n106 = call "Send message to Top.vi"("Data"=w363, "Response"="Module stopped" ("Name"), "Module"=Module_name."Magnet", "Mailbox address in"=w366) -> ()  [unwired: 6 in, 2 out]
      }
      frame "Restart" {
      }
    }
    "PSU Status Out" <- w25
    "Temperatures" <- w28
    "Overall status" <- w26
    "Magnet Constants" <- w30
  }
